vi "ResultToXML.vi"(0 "SN":string, 1 "User":string="root", 5 "FixtureID":string, 7 "EquipmentID":string, 9 "PASS/FAIL?":bool, 11 "Message":T1(array[cluster])) -> (4 "concatenated string":string)   [LabVIEW 2020, in "Salcomp-MES.lvlib" / "CMESAPI.lvclass"]
uses:
  CMESAPI.lvclass
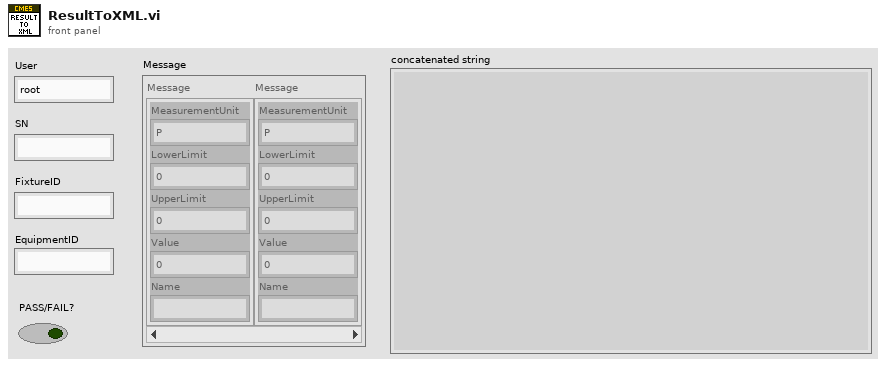
[diagram p1: front panel]
types:
  T1 = cluster{"MeasurementUnit":string, "LowerLimit":string, "UpperLimit":string, "Value":string, "Name":string}[]
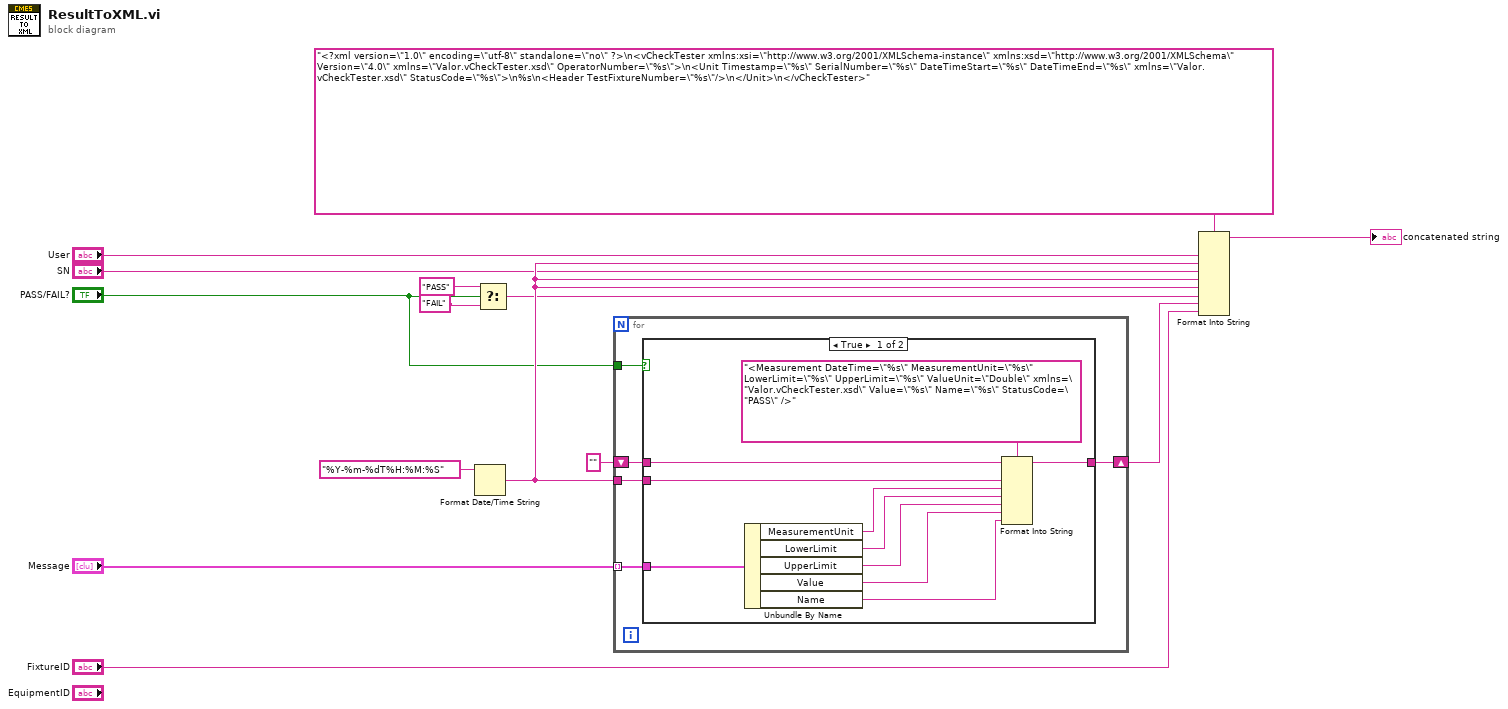
[diagram p0: block diagram]
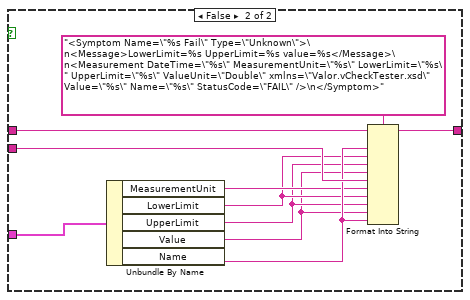
[diagram p2: hidden frame]
diagram:
  n1 = Format Date/Time String(time format string (%c)="%Y-%m-%dT%H:%M:%S") -> (date/time string=w9:string)  [unwired: 2 in]
  n2 = Select(t="PASS", s="PASS/FAIL?", f="FAIL") -> (s? t:f=w8:string)
  n3 = for {
    tunnel: "PASS/FAIL?" -> [w18]
    tunnel: "Message" -> [w17] mode=indexing
    tunnel: w9 -> [w19]
    shift-right: [w15] -> w3
    shift-left: "" -> [w16]
    n4 = case shown="True" w18 {
      tunnel: w17 -> [w26 w36]
      tunnel: w19 -> [w28 w38]
      tunnel: [w27 w37] -> w15
      tunnel: w16 -> [w20 w30]
      frame True {
        n5 = Unbundle By Name(w26) -> ("MeasurementUnit"=w24:string, "LowerLimit"=w23:string, "UpperLimit"=w22:string, "Value"=w21:string, "Name"=w25:string)
        n6 = Format Into String(format string="<Measurement DateTime=\"%s\" MeasurementUnit=\"%s\" LowerLimit=\"%s\" UpperLimit=\"%s\" ValueUnit=\"Double\" xmlns=\"Valor.vCheckTester.xsd\" Value=\"%s\" Name=\"%s\" StatusCode=\"PASS\" />", initial string=w20, w28, w24, w23, w22, w21, w25) -> (resulting string=w27:string)  [unwired: 1 in, 1 out]
      }
      frame False {
        n7 = Unbundle By Name(w36) -> ("MeasurementUnit"=w34:string, "LowerLimit"=w33:string, "UpperLimit"=w32:string, "Value"=w31:string, "Name"=w35:string)
        n8 = Format Into String(format string="<Symptom Name=\"%s Fail\" Type=\"Unknown\">\n<Message>LowerLimit=%s UpperLimit=%s value=%s</Message>\n<Measurement DateTime=\"%s\" MeasurementUnit=\"%s\" LowerLimit=\"%s\" UpperLimit=\"%s\" ValueUnit=\"Double\" xmlns=\"Valor.vCheckTester.xsd\" Value=\"%s\" Name=\"%s\" StatusCode=\"FAIL\" />\n</Symptom>", initial string=w30, w35, w33, w32, w31, w38, w34, w33, w32, w31, w35) -> (resulting string=w37:string)  [unwired: 1 in, 1 out]
      }
    }
  }
  n9 = Format Into String(format string="<?xml version=\"1.0\" encoding=\"utf-8\" standalone=\"no\" ?>\n<vCheckTester xmlns:xsi=\"http://www.w3.org/2001/XMLSchema-instance\" xmlns:xsd=\"http://www.w3.org/2001/XMLSchema\" Version=\"4.0\" xmlns=\"Valor.vCheckTester.xsd\" OperatorNumber=\"%s\">\n<Unit Timestamp=\"%s\" SerialNumber=\"%s\" DateTimeStart=\"%s\" DateTimeEnd=\"%s\" xmlns=\"Valor.vCheckTester.xsd\" StatusCode=\"%s\">\n%s\n<Header TestFixtureNumber=\"%s\"/>\n</Unit>\n</vCheckTester>", "User", w9, "SN", w9, w9, w8, w3, "FixtureID") -> (resulting string=→"concatenated string":string)  [unwired: 2 in, 1 out]
